vi "Sub2.vi"(8 "error in (no error)":errorcluster) -> (0 "error out":errorcluster, 1 "Sun Lat":dbl, 9 "Sun Lon":dbl)   [LabVIEW 2018]
doc: "Use this template to build a VI to use as a subVI. This subVI is getting the sun position In principle, the second VI works the same as the first one, and it has the same front panel and connector design, just with different names for the controls and indicators. It's get the zenith direction of the sun. This\ngives the point on earth were the sun is located 90o vertically above ground."
uses:
  <vilib>/httpClient/LabVIEWHTTPClient.lvlib
panel:
  out "body":string
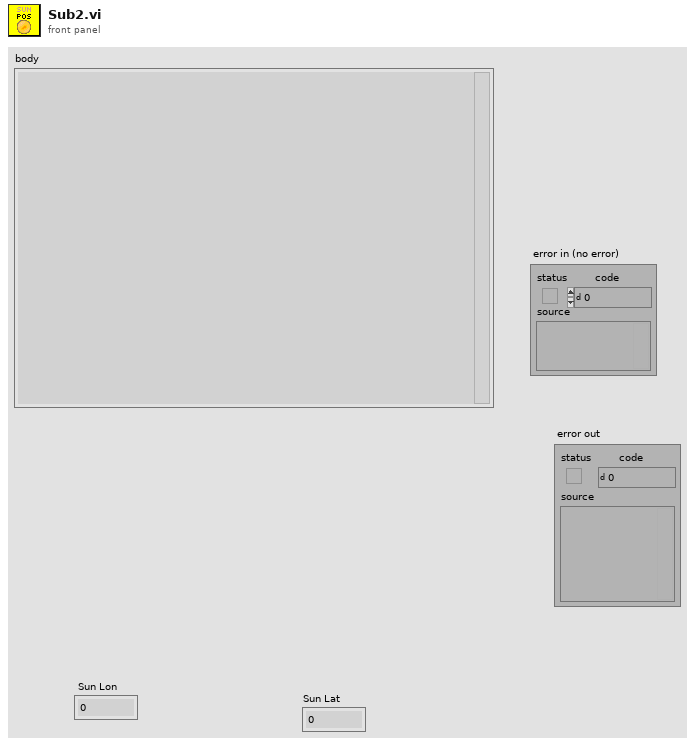
[diagram p1: front panel]
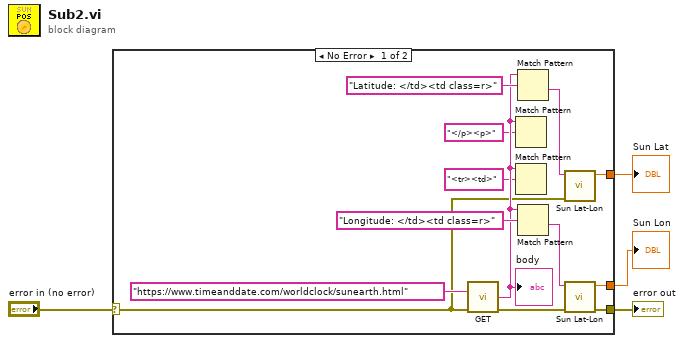
[diagram p0: block diagram]
diagram:
  n1 = case shown="No Error" "error in (no error)" {
    selector: "error in (no error)" -> [w11 w18]
    tunnel: [w9 w18] -> w3
    tunnel: [w8 _] -> w2
    tunnel: [w5 _] -> w1
    frame No Error {
      n2 = call <vilib>:"GET.vi"("url"="https://www.timeanddate.com/worldclock/sunearth.html", "error in (no error)"=w11) -> ("body"=w14:string, "error out"=w10:errorcluster)  [unwired: 10 in, 2 out]
      "body" <- w14
      n3 = Match Pattern(string=w14, regular expression="</p><p>") -> ()  [unwired: 1 in, 4 out]
      n4 = Match Pattern(string=w14, regular expression="<tr><td>") -> ()  [unwired: 1 in, 4 out]
      n5 = Match Pattern(string=w14, regular expression="Latitude: </td><td class=r>") -> (after substring=w6:string)  [unwired: 1 in, 3 out]
      n6 = Match Pattern(string=w14, regular expression="Longitude: </td><td class=r>") -> (after substring=w7:string)  [unwired: 1 in, 3 out]
      n7 = call "Sun Lat-Lon.vi"("error in (no error)"=w11, "Lat/Lon string"=w6) -> ("Converted Position"=w5:dbl)  [unwired: 5 in, 4 out]
      n8 = call "Sun Lat-Lon.vi"("error in (no error)"=w10, "Lat/Lon string"=w7) -> ("error out"=w9:errorcluster, "Converted Position"=w8:dbl)  [unwired: 5 in, 3 out]
    }
    frame Error {
    }
  }
  "error out" <- w3
  "Sun Lat" <- w1
  "Sun Lon" <- w2
